vi "Init PWM.vi"(5 "Phase-Correct (F)":bool, 7 "GPIO #":T1=-1, 8 "error in (no error)":errorcluster, 10 "Enable (F)":bool, 11 "VisaSession in":refnum<class "VisaSession.lvclass">) -> (0 "error out":errorcluster, 2 "PWM":refnum<class "PWM.lvclass">, 3 "VisaSession out":refnum<class "VisaSession.lvclass">)   [LabVIEW 2020, in "CTI.lvlib" / "VisaSession.lvclass"]
uses:
  VisaSession.lvclass
  VisaSession.lvclass/VisaSession.ctl
  Session/Session.lvclass
  PWM/PWM.lvclass
  GPIO Number.ctl
  CTI.lvlib
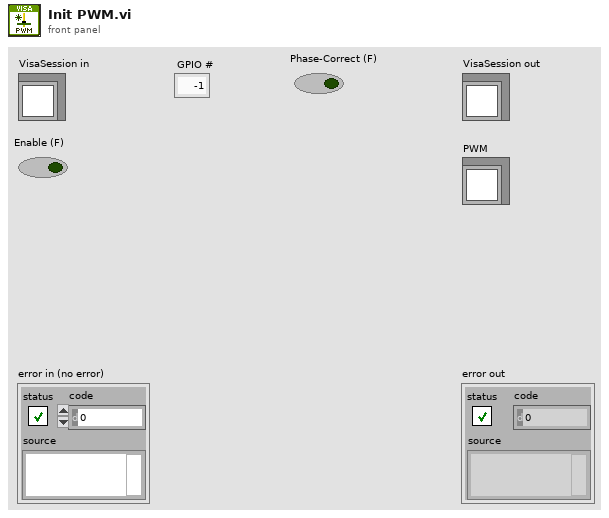
[diagram p1: front panel]
types:
  T1 = typedef "CTI.lvlib/GPIO Number.ctl" = i8
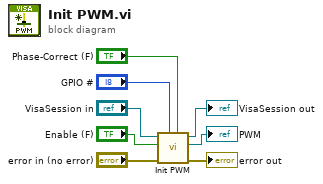
[diagram p0: block diagram]
diagram:
  n1 = call-parent "Init PWM.vi"("Phase-Correct (F)"="Phase-Correct (F)", "GPIO #"="GPIO #", "error in (no error)"="error in (no error)", "Enable (F)"="Enable (F)", "Session in"="VisaSession in") -> ("error out"=→"error out":errorcluster, "PWM"=→"PWM":refnum<class "PWM.lvclass">, "Session out"=→"VisaSession out":refnum<class "VisaSession.lvclass">)  [unwired: 4 in]
